vi "LcWebView_BarPlot_Example.vi"() -> ()   [LabVIEW 2018, in "LcWebView.lvclass"]
doc: "Inject javascript arguments"
uses:
  LcWebView.lvclass
  D:/GitProjects/Public/GitHub/LcWebView/data/Microsoft.Web.WebView2.WinForms.dll
  data/Microsoft.Web.WebView2.WinForms.dll
  plots/ctrls/PlotType.ctl
  plots/ctrls/BarPlotOption.ctl
  plots/ctrls/GenericPlotOption.ctl
  plots/ctrls/LegendPosition.ctl
panel:
  out "BrowserProcessId":u32
  out "Status Message":string
  in  "stop":bool
  in  "Web":refnum<k24>(container)
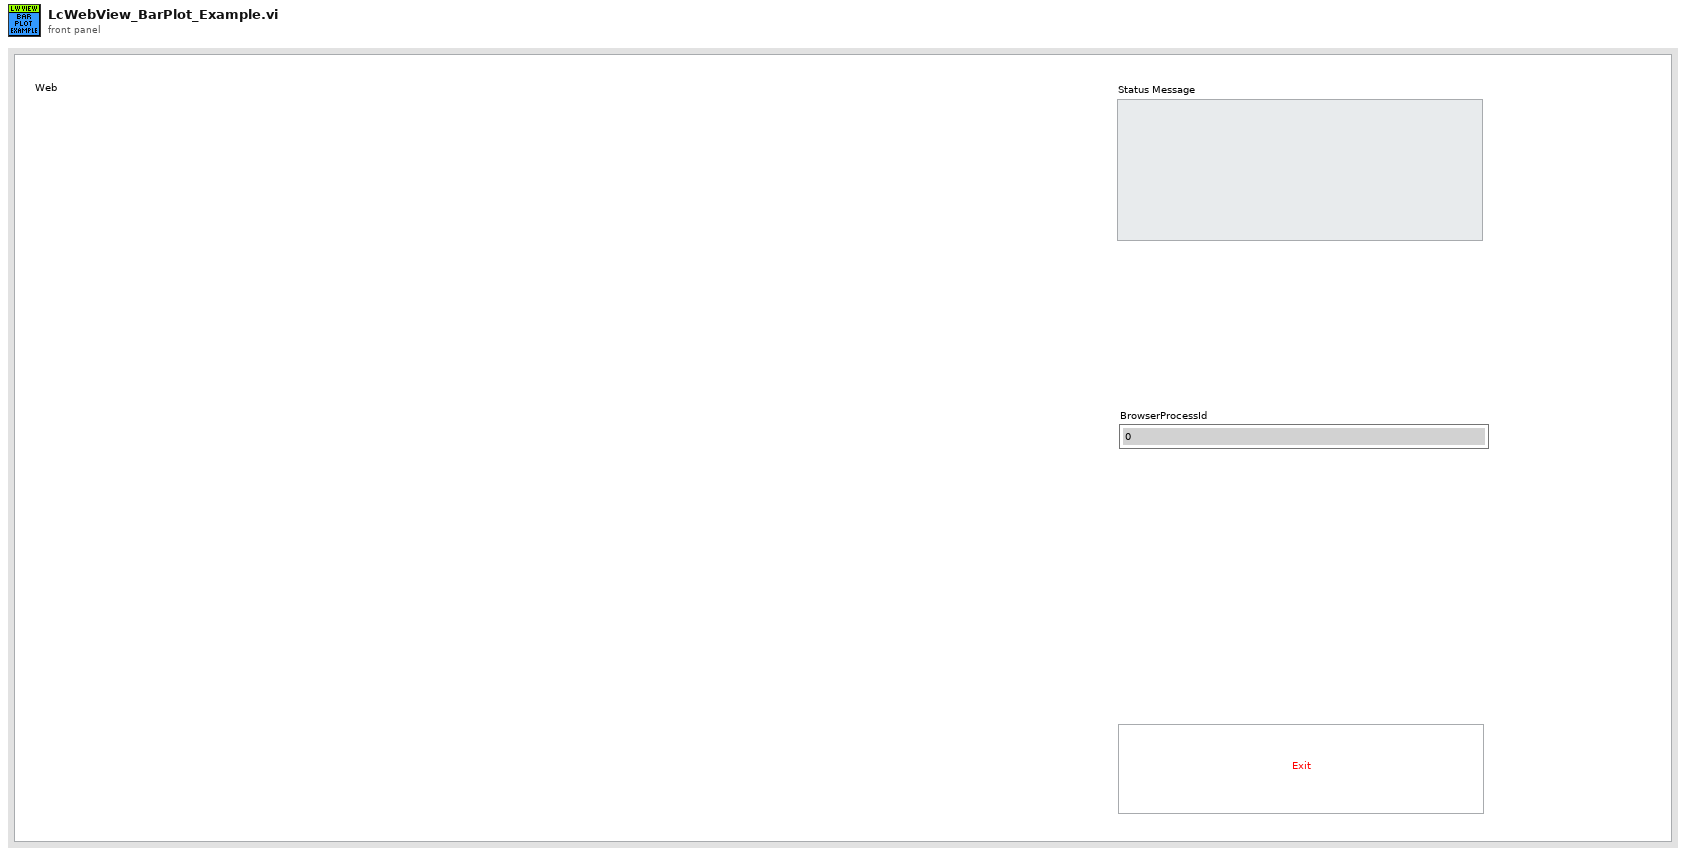
[diagram p1: front panel]
types:
  T1 = typedef "LcWebView.lvclass/GenericPlotOption.ctl" = cluster{"GraphTitle":string, "LegendDisplay":bool, "LegendPosition":T2}
  T2 = typedef "LcWebView.lvclass/LegendPosition.ctl" = enum16{"top", "right", "left", "bottom"}
  T3 = typedef "LcWebView.lvclass/BarPlotOption.ctl" = cluster{"xLabel":string, "yLabel":string, "DisplayXLabel":bool, "DisplayYLabel":bool, "Stacked":bool}
  T4 = typedef "LcWebView.lvclass/PlotType.ctl" = enum16{"bar", "line", "pie", "doughnut", "scatter", "radar", "bubble", "polarArea"}
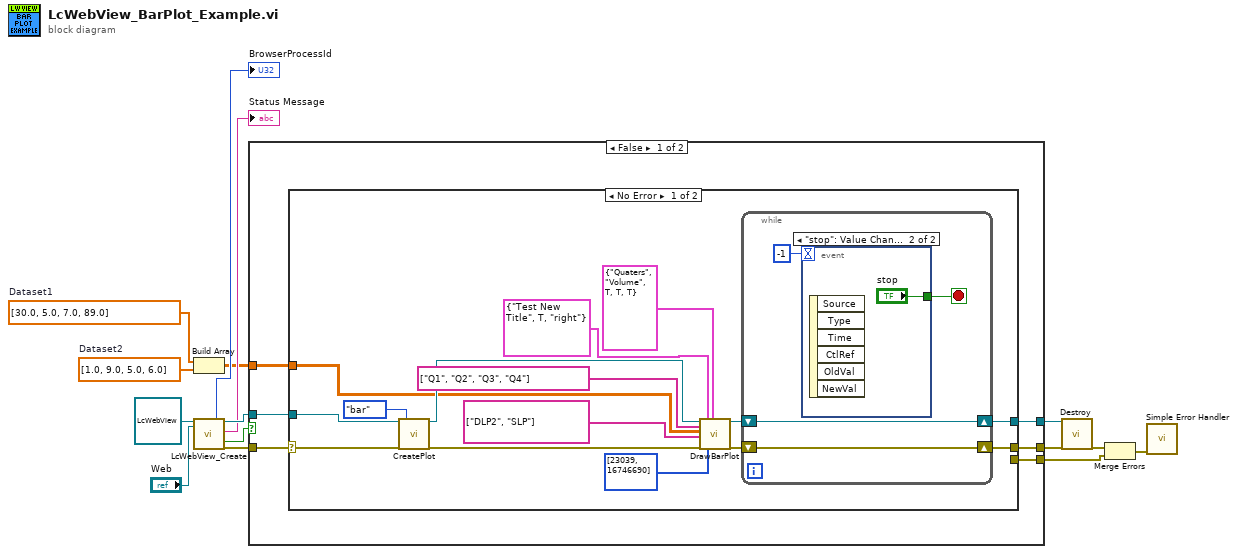
[diagram p0: block diagram]
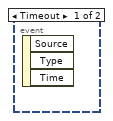
[diagram p2: hidden frame]
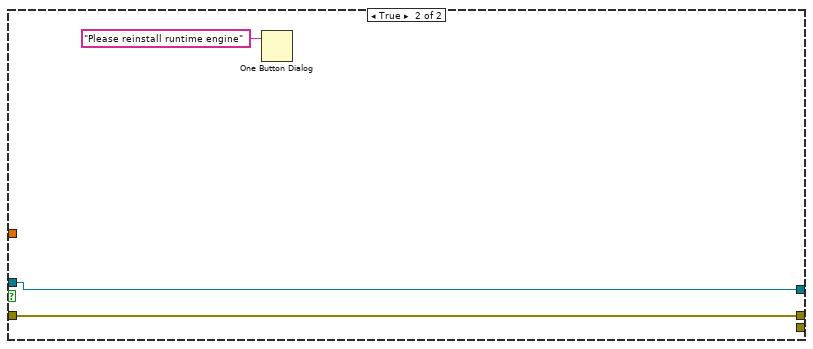
[diagram p4: hidden frame]
diagram:
  w4 = dbl[] [1.0, 9.0, 5.0, 6.0]  # Dataset2
  w3 = dbl[] [30.0, 5.0, 7.0, 89.0]  # Dataset1
  n1 = Build Array(w3, w4) -> (w2:dbl[][])
  n2 = call "LcWebView_Create.vi"("reference in"=refnum<class "LcWebView.lvclass"> refnum, "Webview container"="Web") -> ("BrowserProcessId"=→"BrowserProcessId":u32, "reference out"=w13:refnum<class "LcWebView.lvclass">, "Status Message"=→"Status Message":string, "Reinstall Runtime"=w6:bool, "Error Out"=w12:errorcluster)  [unwired: 10 in, 3 out]
  n3 = case shown="False" w6 {
    tunnel: w13 -> [w21 w46]
    tunnel: w12 -> [w20 w45]
    tunnel: [w19 w46] -> w11
    tunnel: [w17 w45] -> w10
    tunnel: [w18 _] -> w7
    tunnel: w2 -> [w16 _]
    frame False {
      n4 = case shown="No Error" w20 {
        selector: w20 -> [w34 w42]
        tunnel: w21 -> [w35 w43]
        tunnel: [w33 w43] -> w19
        tunnel: [w36 _] -> w17
        tunnel: [_ w42] -> w18
        tunnel: w16 -> [w31 _]
        frame No Error {
          n5 = call-dynamic "CreatePlot.vi"("reference in"=w35, "Error In"=w34, "PlotType"=PlotType."bar") -> ("reference out"=w32:refnum<class "LcWebView.lvclass">, "Error Out"=w28:errorcluster)  [unwired: 15 in]
          n6 = call-dynamic "DrawBarPlot.vi"("reference in"=w32, "XLabels"=string[] ["Q1", "Q2", "Q3", "Q4"], "BarPlot.Dataset"=w31, "BarPlot.DatasetLabels"=string[] ["DLP2", "SLP"] ("DatasetLabels"), "Error In"=w28, "GenericPlotOptions"=T1 {"GraphTitle"="Test New Title", "LegendDisplay"=TRUE, "LegendPosition"=enum."right"}, "BarPlot.PlotColours"=u32[] [23039, 16746690] ("PlotColours"), "BarPlotOptions"=T3 {"xLabel"="Quaters", "yLabel"="Volume", "DisplayXLabel"=TRUE, "DisplayYLabel"=TRUE, "Stacked"=TRUE}) -> ("reference out"=w30:refnum<class "LcWebView.lvclass">, "Error Out"=w29:errorcluster)  [unwired: 10 in]
          n7 = while {
            shift-right: [w40] -> w33
            shift-left: w30 -> [w40]
            shift-right: [w39] -> w36
            shift-left: w29 -> [w39]
            stop <- w37 stop-if-true
            n8 = event shown="[1] \"stop\": Value Change" {
              selector: _ -> [_ _]
              dyn-events: _ -> [_ _]
              timeout: -1 -> [_ _]
              tunnel: [_ "stop"] -> w37
              event Timeout {
                n9 = event-data() -> ()  [unwired: 1 in, 3 out]
              }
              event "stop": Value Change {
                n10 = event-data() -> ()  [unwired: 1 in, 6 out]
              }
            }
          }
        }
        frame Error {
        }
      }
    }
    frame True {
      n11 = One Button Dialog(message="Please reinstall runtime engine") -> ()  [unwired: 1 in, 1 out]
    }
  }
  n12 = call-dynamic "Destroy.vi"("reference in"=w11, "Error In"=w10) -> ("Error Out"=w9:errorcluster)  [unwired: 16 in, 1 out]
  n13 = Merge Errors(w9, w7) -> (w1:errorcluster)
  n14 = call <vilib>:"Simple Error Handler.vi"("error in (no error)"=w1) -> ()  [unwired: 4 in, 5 out]
